vi "Check if IP Port Used.vi"(8 "error in (no error)":errorcluster, 11 "Port":u16) -> (0 "error out":errorcluster, 3 "In Use":bool)   [LabVIEW 2021, in "Networking_CIF_U.lvlib"]
uses:
  Networking_CIF_U.lvlib
  Typedef/Errors.ctl
  Errors/Append Error Location.vi
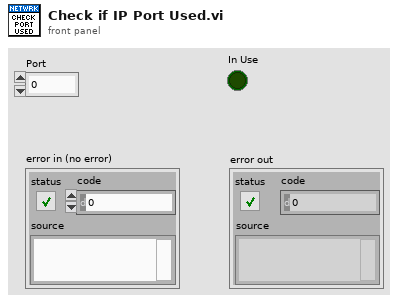
[diagram p1: front panel]
types:
  T1 = typedef "Networking_CIF_U.lvlib/Errors.ctl" = enum16{"Invalid IP Address", "No Subnet Match Found", "Error Finding Port", "No Ping Response", "Nettools Needed", "Error Checking Port"}
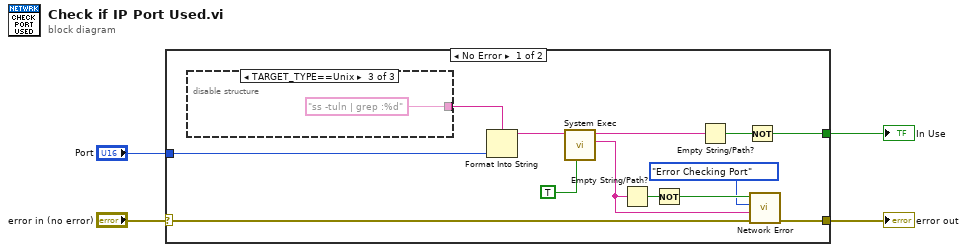
[diagram p0: block diagram]
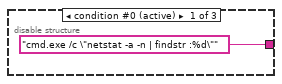
[diagram p2: hidden frame]
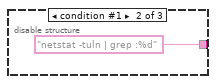
[diagram p3: hidden frame]
diagram:
  n1 = case shown="No Error" "error in (no error)" {
    selector: "error in (no error)" -> [w8 w21]
    tunnel: [w13 w21] -> w4
    tunnel: "Port" -> [w12 _]
    tunnel: [w5 _] -> w1
    frame No Error {
      n2 = disable-structure shown="TARGET_TYPE==Unix" {
        disable-tunnel: ["cmd.exe /c \"netstat -a -n | findstr :%d\"" ("command line") "netstat -tuln | grep :%d" ("command line") "ss -tuln | grep :%d" ("command line")] -> w9
        frame condition #0 (active) {
        }
        frame condition #1 {
        }
        frame condition #2 {
        }
      }
      n3 = Format Into String(format string=w9, w12) -> (resulting string=w11:string)  [unwired: 2 in, 1 out]
      n4 = call <vilib>:"System Exec.vi"("run minimized? (F)"=TRUE, "command line"=w11) -> ("standard error"=w10:string, "standard output"=w7:string)  [unwired: 6 in, 2 out]
      n5 = Empty String/Path?(string/path=w10) -> (empty?=w15:bool)
      n6 = Not(x=w15) -> (.not. x?=w17:bool)
      n7 = Empty String/Path?(string/path=w7) -> (empty?=w6:bool)
      n8 = Not(x=w6) -> (.not. x?=w5:bool)
      n9 = call "Network Error.vi"("error in (no error)"=w8, "String to Append"=w10, "Error"=Errors."Error Checking Port", "Insert Error"=w17) -> ("error out"=w13:errorcluster)  [unwired: 7 in]
    }
    frame Error {
    }
  }
  "error out" <- w4
  "In Use" <- w1
